vi "readLogForceActuatorInfo.vi"(8 "error in (no error)":errorcluster, 10 "Parser":refnum<class "U8ArrayParserAutoIndexing.lvclass">, 11 "M1M3SAL in":refnum<class "M1M3SAL.lvclass">) -> (0 "error out":errorcluster, 2 "EventForceActuatorInfo":variant, 3 "M1M3SAL out":refnum<class "M1M3SAL.lvclass">)   [LabVIEW 2016, in "M1M3SupportCommunicator.lvlib" / "M1M3SAL.lvclass"]
uses:
  M1M3SAL.lvclass
  Common_RT_Utilities/U8ArrayParserAutoIndexing/U8ArrayParserAutoIndexing.lvclass
  DataTypes/Topics/EventForceActuatorInfo.ctl
  DataTypes/Topics/Parts/Timestamp.ctl
  DataTypes/Topics/M1M3SupportTopics.lvlib
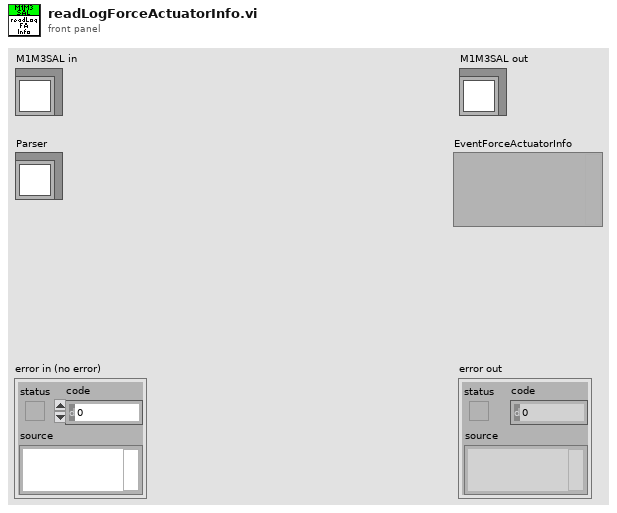
[diagram p1: front panel]
types:
  T1 = typedef "M1M3SupportTopics.lvlib/EventForceActuatorInfo.ctl" = cluster{"Timestamp":T2, "ReferenceId":i32[], "XPosition":sgl[], "YPosition":sgl[], "ZPosition":sgl[], "ILCUniqueId":i64[], "ILCApplicationType":u8[], "NetworkNodeType":u8[], "ILCSelectedOptions":u8[], "NetworkNodeOptions":u8[], "MajorRevision":u8[], "MinorRevision":u8[], "ADCScanRate":u8[], "MainADCCalibrationK1":sgl[], "MainADCCalibrationK2":sgl[], "MainADCCalibrationK3":sgl[], "MainADCCalibrationK4":sgl[], "MainAxialLoadCellOffset":sgl[], "MainLateralLoadCellOffset":sgl[], "MainAxialLoadCellSensitivity":sgl[], "MainLateralLoadCellSensitivity":sgl[], "BackupADCCalibrationK1":sgl[], "BackupADCCalibrationK2":sgl[], "BackupADCCalibrationK3":sgl[], "BackupADCCalibrationK4":sgl[], "BackupAxialLoadCellOffset":sgl[], "BackupLateralLoadCellOffset":sgl[], "BackupAxialLoadCellSensitivity":sgl[], "BackupLateralLoadCellSensitivity":sgl[], "DCAAxialGain":sgl[], "DCALateralGain":sgl[], "DCAUniqueId":i64[], "DCAFirmwareType":u8[], "DCAMajorRevision":u8[], "DCAMinorRevision":u8[], "MainCalibrationError":bool[], "BackupCalibrationError":bool[], "DCAFirmwareUpdate":bool[], "UniqueIdCRCError":bool[], "ApplicationTypeMismatch":bool[], "ApplicationMissing":bool[], "ApplicationCRCMismatch":bool[], "OneWireMissing":bool[], "OneWire1Mismatch":bool[], "OneWire2Mismatch":bool[], "DCAUniqueIdCRCError":bool[], "DCAMainCalibrationError":bool[], "DCABackupCalibrationError":bool[], "DCAApplicationMissing":bool[], "DCAApplicationCRCMismatch":bool[], "DCABootloaderActive":bool[]}
  T2 = typedef "M1M3SupportTopics.lvlib/Timestamp.ctl" = dbl
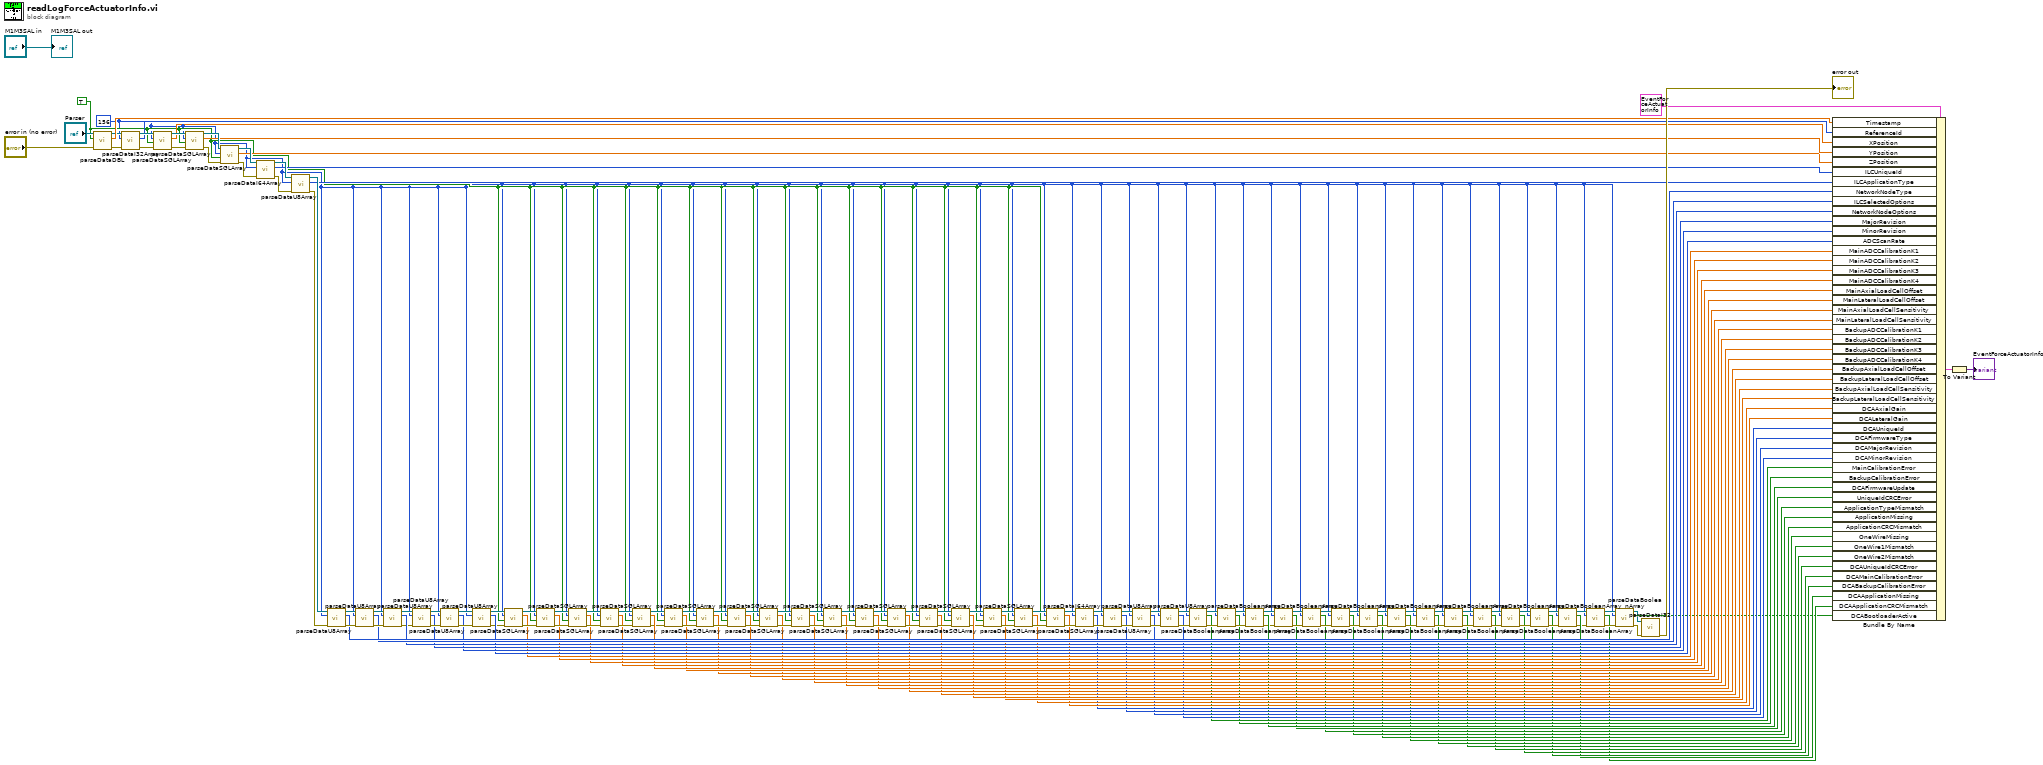
[diagram p0: block diagram]
diagram:
  w1 = 156
  w2 = TRUE ("OverrideSwapBytes")
  n1 = call "parseDataDBL.vi"("error in (no error)"="error in (no error)", "OverrideSwapBytes"=w2, "U8ArrayParserAutoIndexing in"="Parser") -> ("error out"=w3:errorcluster, "Data"=w156:dbl, "U8ArrayParserAutoIndexing out"=w4:refnum<class "U8ArrayParserAutoIndexing.lvclass">)  [unwired: 6 in]
  n2 = call "parseDataI32Array.vi"("U8ArrayParserAutoIndexing in"=w4, "Length"=w1, "error in (no error)"=w3) -> ("U8ArrayParserAutoIndexing out"=w154:refnum<class "U8ArrayParserAutoIndexing.lvclass">, "Data"=w138:i32[], "error out"=w153:errorcluster)  [unwired: 5 in]
  n3 = call "parseDataSGLArray.vi"("U8ArrayParserAutoIndexing in"=w154, "Length"=w1, "OverrideSwapBytes"=w2, "error in (no error)"=w153) -> ("U8ArrayParserAutoIndexing out"=w152:refnum<class "U8ArrayParserAutoIndexing.lvclass">, "Data"=w137:sgl[], "error out"=w151:errorcluster)  [unwired: 4 in]
  n4 = call "parseDataSGLArray.vi"("U8ArrayParserAutoIndexing in"=w152, "Length"=w1, "OverrideSwapBytes"=w2, "error in (no error)"=w151) -> ("U8ArrayParserAutoIndexing out"=w150:refnum<class "U8ArrayParserAutoIndexing.lvclass">, "Data"=w136:sgl[], "error out"=w149:errorcluster)  [unwired: 4 in]
  n5 = call "parseDataSGLArray.vi"("U8ArrayParserAutoIndexing in"=w150, "Length"=w1, "OverrideSwapBytes"=w2, "error in (no error)"=w149) -> ("U8ArrayParserAutoIndexing out"=w148:refnum<class "U8ArrayParserAutoIndexing.lvclass">, "Data"=w135:sgl[], "error out"=w147:errorcluster)  [unwired: 4 in]
  n6 = call "parseDataI64Array.vi"("U8ArrayParserAutoIndexing in"=w148, "Length"=w1, "error in (no error)"=w147) -> ("U8ArrayParserAutoIndexing out"=w146:refnum<class "U8ArrayParserAutoIndexing.lvclass">, "Data"=w134:i64[], "error out"=w145:errorcluster)  [unwired: 5 in]
  n7 = call "parseDataU8Array.vi"("U8ArrayParserAutoIndexing in"=w146, "Length"=w1, "error in (no error)"=w145) -> ("U8ArrayParserAutoIndexing out"=w144:refnum<class "U8ArrayParserAutoIndexing.lvclass">, "Data"=w133:u8[], "error out"=w143:errorcluster)  [unwired: 5 in]
  n8 = call "parseDataU8Array.vi"("U8ArrayParserAutoIndexing in"=w144, "Length"=w1, "error in (no error)"=w143) -> ("U8ArrayParserAutoIndexing out"=w142:refnum<class "U8ArrayParserAutoIndexing.lvclass">, "Data"=w132:u8[], "error out"=w141:errorcluster)  [unwired: 5 in]
  n9 = call "parseDataU8Array.vi"("U8ArrayParserAutoIndexing in"=w142, "Length"=w1, "error in (no error)"=w141) -> ("U8ArrayParserAutoIndexing out"=w140:refnum<class "U8ArrayParserAutoIndexing.lvclass">, "Data"=w131:u8[], "error out"=w139:errorcluster)  [unwired: 5 in]
  n10 = call "parseDataU8Array.vi"("U8ArrayParserAutoIndexing in"=w140, "Length"=w1, "error in (no error)"=w139) -> ("U8ArrayParserAutoIndexing out"=w107:refnum<class "U8ArrayParserAutoIndexing.lvclass">, "Data"=w130:u8[], "error out"=w106:errorcluster)  [unwired: 5 in]
  n11 = call "parseDataU8Array.vi"("U8ArrayParserAutoIndexing in"=w107, "Length"=w1, "error in (no error)"=w106) -> ("U8ArrayParserAutoIndexing out"=w129:refnum<class "U8ArrayParserAutoIndexing.lvclass">, "Data"=w125:u8[], "error out"=w128:errorcluster)  [unwired: 5 in]
  n12 = call "parseDataU8Array.vi"("U8ArrayParserAutoIndexing in"=w129, "Length"=w1, "error in (no error)"=w128) -> ("U8ArrayParserAutoIndexing out"=w127:refnum<class "U8ArrayParserAutoIndexing.lvclass">, "Data"=w124:u8[], "error out"=w126:errorcluster)  [unwired: 5 in]
  n13 = call "parseDataU8Array.vi"("U8ArrayParserAutoIndexing in"=w127, "Length"=w1, "error in (no error)"=w126) -> ("U8ArrayParserAutoIndexing out"=w122:refnum<class "U8ArrayParserAutoIndexing.lvclass">, "Data"=w123:u8[], "error out"=w121:errorcluster)  [unwired: 5 in]
  n14 = call "parseDataSGLArray.vi"("U8ArrayParserAutoIndexing in"=w122, "Length"=w1, "OverrideSwapBytes"=w2, "error in (no error)"=w121) -> ("U8ArrayParserAutoIndexing out"=w118:refnum<class "U8ArrayParserAutoIndexing.lvclass">, "Data"=w112:sgl[], "error out"=w117:errorcluster)  [unwired: 4 in]
  n15 = call "parseDataSGLArray.vi"("U8ArrayParserAutoIndexing in"=w118, "Length"=w1, "OverrideSwapBytes"=w2, "error in (no error)"=w117) -> ("U8ArrayParserAutoIndexing out"=w120:refnum<class "U8ArrayParserAutoIndexing.lvclass">, "Data"=w111:sgl[], "error out"=w119:errorcluster)  [unwired: 4 in]
  n16 = call "parseDataSGLArray.vi"("U8ArrayParserAutoIndexing in"=w120, "Length"=w1, "OverrideSwapBytes"=w2, "error in (no error)"=w119) -> ("U8ArrayParserAutoIndexing out"=w116:refnum<class "U8ArrayParserAutoIndexing.lvclass">, "Data"=w110:sgl[], "error out"=w115:errorcluster)  [unwired: 4 in]
  n17 = call "parseDataSGLArray.vi"("U8ArrayParserAutoIndexing in"=w116, "Length"=w1, "OverrideSwapBytes"=w2, "error in (no error)"=w115) -> ("U8ArrayParserAutoIndexing out"=w114:refnum<class "U8ArrayParserAutoIndexing.lvclass">, "Data"=w109:sgl[], "error out"=w113:errorcluster)  [unwired: 4 in]
  n18 = call "parseDataSGLArray.vi"("U8ArrayParserAutoIndexing in"=w114, "Length"=w1, "OverrideSwapBytes"=w2, "error in (no error)"=w113) -> ("U8ArrayParserAutoIndexing out"=w77:refnum<class "U8ArrayParserAutoIndexing.lvclass">, "Data"=w108:sgl[], "error out"=w76:errorcluster)  [unwired: 4 in]
  n19 = call "parseDataSGLArray.vi"("U8ArrayParserAutoIndexing in"=w77, "Length"=w1, "OverrideSwapBytes"=w2, "error in (no error)"=w76) -> ("U8ArrayParserAutoIndexing out"=w105:refnum<class "U8ArrayParserAutoIndexing.lvclass">, "Data"=w87:sgl[], "error out"=w104:errorcluster)  [unwired: 4 in]
  n20 = call "parseDataSGLArray.vi"("U8ArrayParserAutoIndexing in"=w105, "Length"=w1, "OverrideSwapBytes"=w2, "error in (no error)"=w104) -> ("U8ArrayParserAutoIndexing out"=w103:refnum<class "U8ArrayParserAutoIndexing.lvclass">, "Data"=w86:sgl[], "error out"=w102:errorcluster)  [unwired: 4 in]
  n21 = call "parseDataSGLArray.vi"("U8ArrayParserAutoIndexing in"=w103, "Length"=w1, "OverrideSwapBytes"=w2, "error in (no error)"=w102) -> ("U8ArrayParserAutoIndexing out"=w101:refnum<class "U8ArrayParserAutoIndexing.lvclass">, "Data"=w85:sgl[], "error out"=w100:errorcluster)  [unwired: 4 in]
  n22 = call "parseDataSGLArray.vi"("U8ArrayParserAutoIndexing in"=w101, "Length"=w1, "OverrideSwapBytes"=w2, "error in (no error)"=w100) -> ("U8ArrayParserAutoIndexing out"=w99:refnum<class "U8ArrayParserAutoIndexing.lvclass">, "Data"=w84:sgl[], "error out"=w98:errorcluster)  [unwired: 4 in]
  n23 = call "parseDataSGLArray.vi"("U8ArrayParserAutoIndexing in"=w99, "Length"=w1, "OverrideSwapBytes"=w2, "error in (no error)"=w98) -> ("U8ArrayParserAutoIndexing out"=w97:refnum<class "U8ArrayParserAutoIndexing.lvclass">, "Data"=w83:sgl[], "error out"=w96:errorcluster)  [unwired: 4 in]
  n24 = call "parseDataSGLArray.vi"("U8ArrayParserAutoIndexing in"=w97, "Length"=w1, "OverrideSwapBytes"=w2, "error in (no error)"=w96) -> ("U8ArrayParserAutoIndexing out"=w95:refnum<class "U8ArrayParserAutoIndexing.lvclass">, "Data"=w82:sgl[], "error out"=w94:errorcluster)  [unwired: 4 in]
  n25 = call "parseDataSGLArray.vi"("U8ArrayParserAutoIndexing in"=w95, "Length"=w1, "OverrideSwapBytes"=w2, "error in (no error)"=w94) -> ("U8ArrayParserAutoIndexing out"=w93:refnum<class "U8ArrayParserAutoIndexing.lvclass">, "Data"=w81:sgl[], "error out"=w92:errorcluster)  [unwired: 4 in]
  n26 = call "parseDataSGLArray.vi"("U8ArrayParserAutoIndexing in"=w93, "Length"=w1, "OverrideSwapBytes"=w2, "error in (no error)"=w92) -> ("U8ArrayParserAutoIndexing out"=w91:refnum<class "U8ArrayParserAutoIndexing.lvclass">, "Data"=w80:sgl[], "error out"=w90:errorcluster)  [unwired: 4 in]
  n27 = call "parseDataSGLArray.vi"("U8ArrayParserAutoIndexing in"=w91, "Length"=w1, "OverrideSwapBytes"=w2, "error in (no error)"=w90) -> ("U8ArrayParserAutoIndexing out"=w89:refnum<class "U8ArrayParserAutoIndexing.lvclass">, "Data"=w79:sgl[], "error out"=w88:errorcluster)  [unwired: 4 in]
  n28 = call "parseDataSGLArray.vi"("U8ArrayParserAutoIndexing in"=w89, "Length"=w1, "OverrideSwapBytes"=w2, "error in (no error)"=w88) -> ("U8ArrayParserAutoIndexing out"=w47:refnum<class "U8ArrayParserAutoIndexing.lvclass">, "Data"=w78:sgl[], "error out"=w46:errorcluster)  [unwired: 4 in]
  n29 = call "parseDataSGLArray.vi"("U8ArrayParserAutoIndexing in"=w47, "Length"=w1, "OverrideSwapBytes"=w2, "error in (no error)"=w46) -> ("U8ArrayParserAutoIndexing out"=w75:refnum<class "U8ArrayParserAutoIndexing.lvclass">, "Data"=w57:sgl[], "error out"=w74:errorcluster)  [unwired: 4 in]
  n30 = call "parseDataSGLArray.vi"("U8ArrayParserAutoIndexing in"=w75, "Length"=w1, "OverrideSwapBytes"=w2, "error in (no error)"=w74) -> ("U8ArrayParserAutoIndexing out"=w73:refnum<class "U8ArrayParserAutoIndexing.lvclass">, "Data"=w56:sgl[], "error out"=w72:errorcluster)  [unwired: 4 in]
  n31 = call "parseDataSGLArray.vi"("U8ArrayParserAutoIndexing in"=w73, "Length"=w1, "OverrideSwapBytes"=w2, "error in (no error)"=w72) -> ("U8ArrayParserAutoIndexing out"=w71:refnum<class "U8ArrayParserAutoIndexing.lvclass">, "Data"=w55:sgl[], "error out"=w70:errorcluster)  [unwired: 4 in]
  n32 = call "parseDataI64Array.vi"("U8ArrayParserAutoIndexing in"=w71, "Length"=w1, "error in (no error)"=w70) -> ("U8ArrayParserAutoIndexing out"=w69:refnum<class "U8ArrayParserAutoIndexing.lvclass">, "Data"=w54:i64[], "error out"=w68:errorcluster)  [unwired: 5 in]
  n33 = call "parseDataU8Array.vi"("U8ArrayParserAutoIndexing in"=w69, "Length"=w1, "error in (no error)"=w68) -> ("U8ArrayParserAutoIndexing out"=w67:refnum<class "U8ArrayParserAutoIndexing.lvclass">, "Data"=w53:u8[], "error out"=w66:errorcluster)  [unwired: 5 in]
  n34 = call "parseDataU8Array.vi"("U8ArrayParserAutoIndexing in"=w67, "Length"=w1, "error in (no error)"=w66) -> ("U8ArrayParserAutoIndexing out"=w65:refnum<class "U8ArrayParserAutoIndexing.lvclass">, "Data"=w52:u8[], "error out"=w64:errorcluster)  [unwired: 5 in]
  n35 = call "parseDataU8Array.vi"("U8ArrayParserAutoIndexing in"=w65, "Length"=w1, "error in (no error)"=w64) -> ("U8ArrayParserAutoIndexing out"=w62:refnum<class "U8ArrayParserAutoIndexing.lvclass">, "Data"=w51:u8[], "error out"=w63:errorcluster)  [unwired: 5 in]
  n36 = call "parseDataBooleanArray.vi"("error in (no error)"=w63, "Length"=w1, "U8ArrayParserAutoIndexing in"=w62) -> ("error out"=w61:errorcluster, "Data"=w50:bool[], "U8ArrayParserAutoIndexing out"=w60:refnum<class "U8ArrayParserAutoIndexing.lvclass">)  [unwired: 6 in]
  n37 = call "parseDataBooleanArray.vi"("error in (no error)"=w61, "Length"=w1, "U8ArrayParserAutoIndexing in"=w60) -> ("error out"=w59:errorcluster, "Data"=w49:bool[], "U8ArrayParserAutoIndexing out"=w58:refnum<class "U8ArrayParserAutoIndexing.lvclass">)  [unwired: 6 in]
  n38 = call "parseDataBooleanArray.vi"("error in (no error)"=w59, "Length"=w1, "U8ArrayParserAutoIndexing in"=w58) -> ("error out"=w7:errorcluster, "Data"=w48:bool[], "U8ArrayParserAutoIndexing out"=w8:refnum<class "U8ArrayParserAutoIndexing.lvclass">)  [unwired: 6 in]
  n39 = call "parseDataBooleanArray.vi"("error in (no error)"=w7, "Length"=w1, "U8ArrayParserAutoIndexing in"=w8) -> ("error out"=w45:errorcluster, "Data"=w25:bool[], "U8ArrayParserAutoIndexing out"=w44:refnum<class "U8ArrayParserAutoIndexing.lvclass">)  [unwired: 6 in]
  n40 = call "parseDataBooleanArray.vi"("error in (no error)"=w45, "Length"=w1, "U8ArrayParserAutoIndexing in"=w44) -> ("error out"=w43:errorcluster, "Data"=w24:bool[], "U8ArrayParserAutoIndexing out"=w42:refnum<class "U8ArrayParserAutoIndexing.lvclass">)  [unwired: 6 in]
  n41 = call "parseDataBooleanArray.vi"("error in (no error)"=w43, "Length"=w1, "U8ArrayParserAutoIndexing in"=w42) -> ("error out"=w41:errorcluster, "Data"=w23:bool[], "U8ArrayParserAutoIndexing out"=w40:refnum<class "U8ArrayParserAutoIndexing.lvclass">)  [unwired: 6 in]
  n42 = call "parseDataBooleanArray.vi"("error in (no error)"=w41, "Length"=w1, "U8ArrayParserAutoIndexing in"=w40) -> ("error out"=w39:errorcluster, "Data"=w22:bool[], "U8ArrayParserAutoIndexing out"=w38:refnum<class "U8ArrayParserAutoIndexing.lvclass">)  [unwired: 6 in]
  n43 = call "parseDataBooleanArray.vi"("error in (no error)"=w39, "Length"=w1, "U8ArrayParserAutoIndexing in"=w38) -> ("error out"=w27:errorcluster, "Data"=w21:bool[], "U8ArrayParserAutoIndexing out"=w29:refnum<class "U8ArrayParserAutoIndexing.lvclass">)  [unwired: 6 in]
  n44 = call "parseDataBooleanArray.vi"("error in (no error)"=w27, "Length"=w1, "U8ArrayParserAutoIndexing in"=w29) -> ("error out"=w26:errorcluster, "Data"=w20:bool[], "U8ArrayParserAutoIndexing out"=w28:refnum<class "U8ArrayParserAutoIndexing.lvclass">)  [unwired: 6 in]
  n45 = call "parseDataBooleanArray.vi"("error in (no error)"=w26, "Length"=w1, "U8ArrayParserAutoIndexing in"=w28) -> ("error out"=w37:errorcluster, "Data"=w19:bool[], "U8ArrayParserAutoIndexing out"=w36:refnum<class "U8ArrayParserAutoIndexing.lvclass">)  [unwired: 6 in]
  n46 = call "parseDataBooleanArray.vi"("error in (no error)"=w37, "Length"=w1, "U8ArrayParserAutoIndexing in"=w36) -> ("error out"=w35:errorcluster, "Data"=w18:bool[], "U8ArrayParserAutoIndexing out"=w34:refnum<class "U8ArrayParserAutoIndexing.lvclass">)  [unwired: 6 in]
  n47 = call "parseDataBooleanArray.vi"("error in (no error)"=w35, "Length"=w1, "U8ArrayParserAutoIndexing in"=w34) -> ("error out"=w33:errorcluster, "Data"=w17:bool[], "U8ArrayParserAutoIndexing out"=w32:refnum<class "U8ArrayParserAutoIndexing.lvclass">)  [unwired: 6 in]
  n48 = call "parseDataBooleanArray.vi"("error in (no error)"=w33, "Length"=w1, "U8ArrayParserAutoIndexing in"=w32) -> ("error out"=w31:errorcluster, "Data"=w16:bool[], "U8ArrayParserAutoIndexing out"=w30:refnum<class "U8ArrayParserAutoIndexing.lvclass">)  [unwired: 6 in]
  n49 = call "parseDataBooleanArray.vi"("error in (no error)"=w31, "Length"=w1, "U8ArrayParserAutoIndexing in"=w30) -> ("error out"=w9:errorcluster, "Data"=w15:bool[], "U8ArrayParserAutoIndexing out"=w10:refnum<class "U8ArrayParserAutoIndexing.lvclass">)  [unwired: 6 in]
  n50 = call "parseDataBooleanArray.vi"("error in (no error)"=w9, "Length"=w1, "U8ArrayParserAutoIndexing in"=w10) -> ("error out"=w14:errorcluster, "Data"=w12:bool[], "U8ArrayParserAutoIndexing out"=w13:refnum<class "U8ArrayParserAutoIndexing.lvclass">)  [unwired: 6 in]
  n51 = call "parseDataBooleanArray.vi"("error in (no error)"=w14, "Length"=w1, "U8ArrayParserAutoIndexing in"=w13) -> ("error out"=w5:errorcluster, "Data"=w11:bool[], "U8ArrayParserAutoIndexing out"=w6:refnum<class "U8ArrayParserAutoIndexing.lvclass">)  [unwired: 6 in]
  n52 = call "parseDataI32.vi"("error in (no error)"=w5, "U8ArrayParserAutoIndexing in"=w6) -> ("error out"=→"error out":errorcluster)  [unwired: 7 in, 2 out]
  n53 = Bundle By Name(cluster=T1 {"Timestamp"=0.0, "ReferenceId"=[], "XPosition"=[], "YPosition"=[], "ZPosition"=[], "ILCUniqueId"=[], "ILCApplicationType"=[], "NetworkNodeType"=[], "ILCSelectedOptions"=[], "NetworkNodeOptions"=[], "MajorRevision"=[], "MinorRevision"=[], "ADCScanRate"=[], "MainADCCalibrationK1"=[], "MainADCCalibrationK2"=[], "MainADCCalibrationK3"=[], "MainADCCalibrationK4"=[], "MainAxialLoadCellOffset"=[], "MainLateralLoadCellOffset"=[], "MainAxialLoadCellSensitivity"=[], "MainLateralLoadCellSensitivity"=[], "BackupADCCalibrationK1"=[], "BackupADCCalibrationK2"=[], "BackupADCCalibrationK3"=[], "BackupADCCalibrationK4"=[], "BackupAxialLoadCellOffset"=[], "BackupLateralLoadCellOffset"=[], "BackupAxialLoadCellSensitivity"=[], "BackupLateralLoadCellSensitivity"=[], "DCAAxialGain"=[], "DCALateralGain"=[], "DCAUniqueId"=[], "DCAFirmwareType"=[], "DCAMajorRevision"=[], "DCAMinorRevision"=[], "MainCalibrationError"=[], "BackupCalibrationError"=[], "DCAFirmwareUpdate"=[], "UniqueIdCRCError"=[], "ApplicationTypeMismatch"=[], "ApplicationMissing"=[], "ApplicationCRCMismatch"=[], "OneWireMissing"=[], "OneWire1Mismatch"=[], "OneWire2Mismatch"=[], "DCAUniqueIdCRCError"=[], "DCAMainCalibrationError"=[], "DCABackupCalibrationError"=[], "DCAApplicationMissing"=[], "DCAApplicationCRCMismatch"=[], "DCABootloaderActive"=[]} ("EventForceActuatorInfo"), "Timestamp"=w156, "ReferenceId"=w138, "XPosition"=w137, "YPosition"=w136, "ZPosition"=w135, "ILCUniqueId"=w134, "ILCApplicationType"=w133, "NetworkNodeType"=w132, "ILCSelectedOptions"=w131, "NetworkNodeOptions"=w130, "MajorRevision"=w125, "MinorRevision"=w124, "ADCScanRate"=w123, "MainADCCalibrationK1"=w112, "MainADCCalibrationK2"=w111, "MainADCCalibrationK3"=w110, "MainADCCalibrationK4"=w109, "MainAxialLoadCellOffset"=w108, "MainLateralLoadCellOffset"=w87, "MainAxialLoadCellSensitivity"=w86, "MainLateralLoadCellSensitivity"=w85, "BackupADCCalibrationK1"=w84, "BackupADCCalibrationK2"=w83, "BackupADCCalibrationK3"=w82, "BackupADCCalibrationK4"=w81, "BackupAxialLoadCellOffset"=w80, "BackupLateralLoadCellOffset"=w79, "BackupAxialLoadCellSensitivity"=w78, "BackupLateralLoadCellSensitivity"=w57, "DCAAxialGain"=w56, "DCALateralGain"=w55, "DCAUniqueId"=w54, "DCAFirmwareType"=w53, "DCAMajorRevision"=w52, "DCAMinorRevision"=w51, "MainCalibrationError"=w50, "BackupCalibrationError"=w49, "DCAFirmwareUpdate"=w48, "UniqueIdCRCError"=w25, "ApplicationTypeMismatch"=w24, "ApplicationMissing"=w23, "ApplicationCRCMismatch"=w22, "OneWireMissing"=w21, "OneWire1Mismatch"=w20, "OneWire2Mismatch"=w19, "DCAUniqueIdCRCError"=w18, "DCAMainCalibrationError"=w17, "DCABackupCalibrationError"=w16, "DCAApplicationMissing"=w15, "DCAApplicationCRCMismatch"=w12, "DCABootloaderActive"=w11) -> (w161:T1)
  n54 = To Variant(anything=w161) -> (Variant=→"EventForceActuatorInfo":variant)
  "M1M3SAL out" <- "M1M3SAL in"
